vi "GetXL_CellValues_2D_String.vi"(8 "error in":errorcluster, 9 "End":cluster{"Column":i32, "Row":i32}, 10 "Start":cluster{"Column":i32, "Row":i32}, 11 "Refnum Cluster In":T1) -> (0 "error out":errorcluster, 2 "data":string[][](array[string]), 3 "Refnum Cluster Out":T1)   [LabVIEW 2015]
doc: "This VI returns the value of a range of cells starting at a given row and column and ending at a given row and column.\n\nThe output data is in variant form and must be converted to string or numeric format."
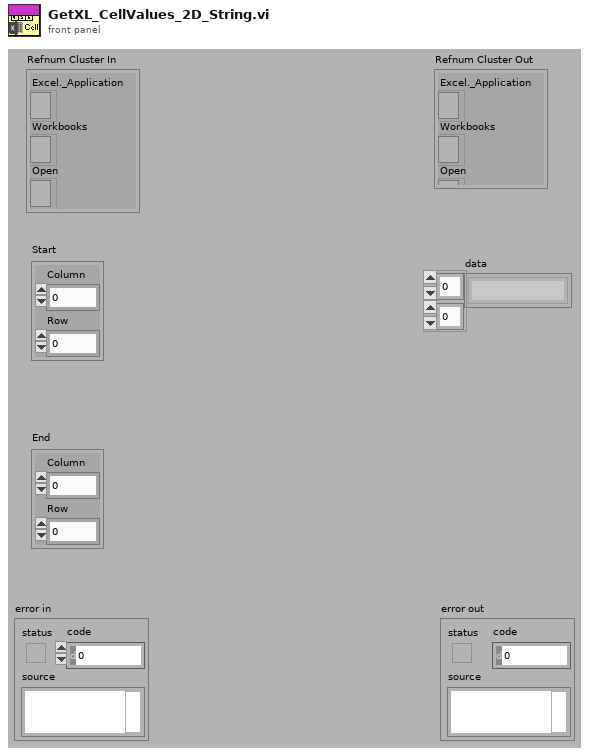
[diagram p1: front panel]
types:
  T1 = cluster{"Excel._Application":refnum<k7>, "Workbooks":refnum<k7>, "Open":refnum<k7>, "Worksheets":refnum<k7>, "Excel._Worksheet":refnum<k7>}
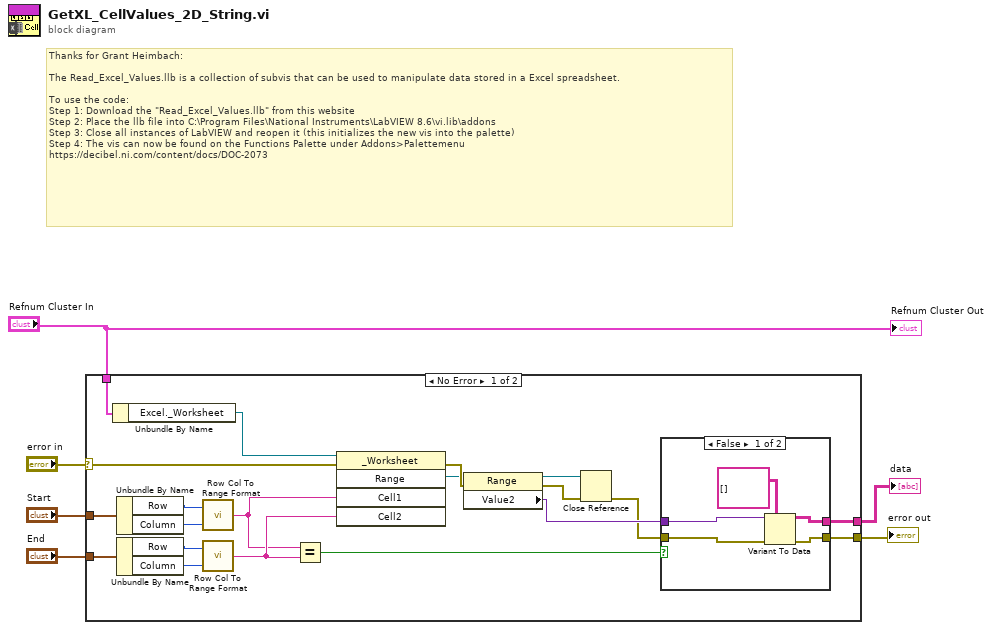
[diagram p0: block diagram]
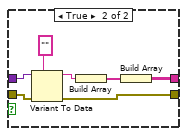
[diagram p2: hidden frame]
diagram:
  # "Thanks for Grant Heimbach: \n\nThe Read_Excel_Values.llb is a collection of subvis that can be used to manipulate data stored in a Excel spreadsheet.\n \nTo use the code:\nStep 1: Download the \"Read_Excel_Values.llb\" from this website\nStep 2: Place the llb file into C:\\Program Files\\National Instruments\\LabVIEW 8.6\\vi.lib\\addons\nStep 3: Close all instances of LabVIEW and reopen it (this initializes the new vis into the palette)\nStep 4: The vis can now be found on the Functions Palette under Addons>Palettemenu\nhttps://decibel.ni.com/content/docs/DOC-2073"
  n1 = case shown="No Error" "error in" {
    selector: "error in" -> [w26 w39]
    tunnel: "Start" -> [w21 _]
    tunnel: "End" -> [w18 _]
    tunnel: [w13 w39] -> w3
    tunnel: [w12 _] -> w2
    tunnel: "Refnum Cluster In" -> [w8 _]
    frame No Error {
      n2 = Unbundle By Name(w8) -> ("Excel._Worksheet"=w7:refnum<k7>)
      n3 = Unbundle By Name(w21) -> ("Row"=w20:i32, "Column"=w19:i32)
      n4 = Unbundle By Name(w18) -> ("Row"=w17:i32, "Column"=w16:i32)
      n5 = call "Row Col To Range Format.vi"("Column"=w19, "Row"=w20) -> ("Output String"=w10:string)
      n6 = call "Row Col To Range Format.vi"("Column"=w16, "Row"=w17) -> ("Output String"=w11:string)
      n7 = Equal?(x=w10, y=w11) -> (x = y?=w9:bool)
      n8 = invoke class="_Worksheet" method="Range"(reference=w7, error in=w26, "Cell1"=w10, "Cell2"=w11) -> (error out=w25:errorcluster, "Range"=w24:refnum<k7>)  [unwired: 1 in, 3 out]
      n9 = property class="Range"(reference=w24, error in=w25) -> (reference out=w23:refnum<k7>, error out=w22:errorcluster, "Value2"=w15:variant)
      n10 = Close Reference(reference=w23, error in (no error)=w22) -> (error out=w14:errorcluster)
      n11 = case shown="False" w9 {
        tunnel: w15 -> [w31 w37]
        tunnel: w14 -> [w30 w38]
        tunnel: [w29 w36] -> w13
        tunnel: [w27 w32] -> w12
        frame False {
          n12 = Variant To Data(error in=w30, type=string[][] [], Variant=w31) -> (data=w27:string[][], error out=w29:errorcluster)
        }
        frame True {
          n13 = Variant To Data(error in=w38, type="", Variant=w37) -> (data=w34:string, error out=w36:errorcluster)
          n14 = Build Array(w34) -> (w33:string[])
          n15 = Build Array(w33) -> (w32:string[][])
        }
      }
    }
    frame Error {
    }
  }
  "error out" <- w3
  "data" <- w2
  "Refnum Cluster Out" <- "Refnum Cluster In"
